vi "SetLimit.vi"(1 "MaxRange":dbl format="%.2f", 2 "MinRange":dbl format="%.2f", 3 "DLL path in":path, 4 "Axis":i32=1) -> (0 "error out":errorcluster)   [LabVIEW 2015, in "DelayLineLS4.lvclass"]
uses:
  Classes/Delay Line/DelayLineLS4/DelayLineLS4.lvclass
  <vilib>/Utility/error.llb/DialogType.ctl
  <vilib>/ErrorRing/Error Ring.xnode
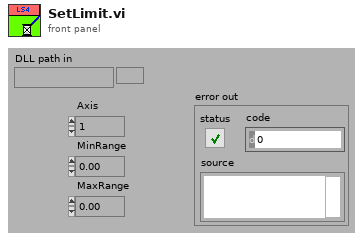
[diagram p1: front panel]
types:
  T1 = typedef "DialogType.ctl" = u16
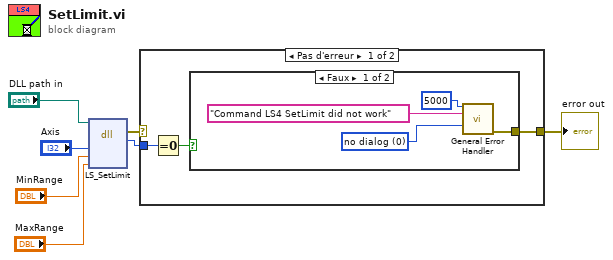
[diagram p0: block diagram]
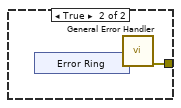
[diagram p2: hidden frame]
diagram:
  n1 = dll-call lib="LStep4.dll" fn="LS_SetLimit"(path in="DLL path in", "Axis"="Axis", "MinRange"="MinRange", "MaxRange"="MaxRange") -> (error out=w2:errorcluster, "type de retour"=w7:i32)  [unwired: 5 in, 1 out]
  n2 = case shown="Pas d'erreur" w2 {
    selector: w2 -> [_ w18]
    tunnel: w7 -> [w10 _]
    tunnel: [w9 w18] -> w3
    frame No Error {
      n3 = Equal To 0?(x=w10) -> (x = 0?=w8:bool)
      n4 = case shown="Faux" w8 {
        tunnel: [w12 w15] -> w9
        frame False {
          w11 = T1 0 items=["no dialog", "OK message", "continue or stop message", "OK message + warnings", "continue/stop + warnings"] ("type of dialog (OK msg:1)")
          n5 = call <vilib>:"General Error Handler.vi"("[error code] (0)"=5000 ("code"), "[error source] (\" \")"="Command LS4 SetLimit did not work" ("String to Prepend to source (\"\")"), "type of dialog (OK msg:1)"=w11) -> ("error out"=w12:errorcluster)  [unwired: 8 in, 4 out]
        }
        frame True {
          n6 = xnode "Error Ring"() -> ("sortie d'erreur"=w16:errorcluster)
          n7 = call <vilib>:"General Error Handler.vi"("error in (no error)"=w16) -> ("error out"=w15:errorcluster)  [unwired: 10 in, 4 out]
        }
      }
    }
    frame Error {
    }
  }
  "error out" <- w3
